vi "ConfigureDAQ.vi"(11 "DAQ Config Data":T1={"Vertical"={"Coupling"=0, "Offset (V)"=0.0, "Range (V)"=0.0, "Impedance"=0.0}, "Horizontal"={"Offset Time"=0.0, "Sample Time (S)"=0.0, "Sample Points"=0}, "Trigger\n"={"Lower Level (V)"=0.0, "Trigger Slope"=0, "Trigger Source"=0}, "Acquisition"={"Trigger Mode"=0, "Initiate Continuously"=0, "Acquire Type"=0, "Acquire Count"=1}, "Channel"=0, "Instrument Handle"=0, "Error"={"status"=FALSE, "code"=0, "source"=""}, "State"=0} {"State" items=["Enable"=1, "Disable"=0]; "Channel" items=["Input Channel 1", "Input Channel 2", "Input Channel 3", "Input Channel 4"]; "Acquisition"."Acquire Type" items=["Normal"=0, "Average"=1, "Envelope"=2, "Peak Detect"=3, "High Resolution"=4, "Fast"=5, "Equivalent Time"=16]; "Acquisition"."Initiate Continuously" items=["Continuously"=1, "Single Capture"=0]; "Acquisition"."Trigger Mode" items=["Auto", "Normal"]; "Trigger"."Trigger Source" items=["TTL0", "TTL1", "TTL2", "TTL3", "TTL4", "TTL5", "TTL6", "TTL7", "ECL0", "ECL1", "Input Channel 1", "Input Channel 2", "Input Channel 3", "Input Channel 4", "External Trigger Source", "STAR", "Manual Trigger", "Pattern"]; "Trigger"."Trigger Slope" items=["Rising Edge", "Falling Edge"]; "Horizontal"."Sample Time (S)" items=["0.5"=0.5, "0.4"=0.4, "0.25"=0.25, "0.2"=0.2, "0.1"=0.1, "0.05"=0.05, "0.04"=0.04, "0.025"=0.025, "0.02"=0.02, "0.01"=0.01, "0.005"=0.005, "0.004"=0.004, "0.0025"=0.0025, "0.002"=0.002, "0.001"=0.001, "5E-4"=0.0005, "4E-4"=0.0004, "2.5E-4"=0.00025, "2E-4"=0.0002, "1E-4"=0.0001, "5E-5"=5e-05, "4E-5"=4e-05, "2E-5"=2e-05, "5E-6"=5e-06, "1E-6"=1e-06, "5E-7"=5e-07, "1E-7"=1e-07, "5E-8"=5e-08, "1E-8"=1e-08]; "Vertical"."Impedance" items=["50 Ohm"=50.0, "1 MOhm"=1000000.0]; "Vertical"."Range (V)" items=["10"=10.0, "5"=5.0, "2"=2.0, "1"=1.0, "0.4"=0.4, "0.2"=0.2, "0.08"=0.08, "0.04"=0.04, "0.02"=0.02, "0.01"=0.01]; "Vertical"."Coupling" items=["AC", "DC"]}) -> (0 "error out":errorcluster, 3 "Instrument Handle Out":i32)   [LabVIEW 2023]
uses:
  TypeDefs/DataTypes/DAQConfig.ctl
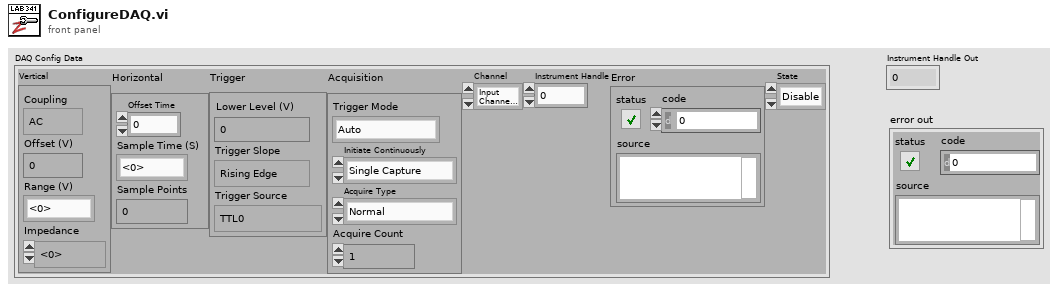
[diagram p1: front panel]
types:
  T1 = typedef "DAQConfig.ctl" = cluster{"Vertical":cluster{"Coupling":i32, "Offset (V)":dbl, "Range (V)":dbl, "Impedance":dbl}, "Horizontal":cluster{"Offset Time":dbl, "Sample Time (S)":dbl, "Sample Points":u32}, "Trigger\n":cluster{"Lower Level (V)":dbl, "Trigger Slope":i32, "Trigger Source":i32}, "Acquisition":cluster{"Trigger Mode":i32, "Initiate Continuously":i32, "Acquire Type":i32, "Acquire Count":i32}, "Channel":i32, "Instrument Handle":i32, "Error":errorcluster, "State":i32}
  T2 = cluster{"Lower Level (V)":dbl, "Trigger Slope":i32, "Trigger Source":i32}
  T3 = cluster{"Trigger Mode":i32, "Initiate Continuously":i32, "Acquire Type":i32, "Acquire Count":i32}
  T4 = cluster{"Coupling":i32, "Offset (V)":dbl, "Range (V)":dbl, "Impedance":dbl}
  T5 = cluster{"Offset Time":dbl, "Sample Time (S)":dbl, "Sample Points":u32}
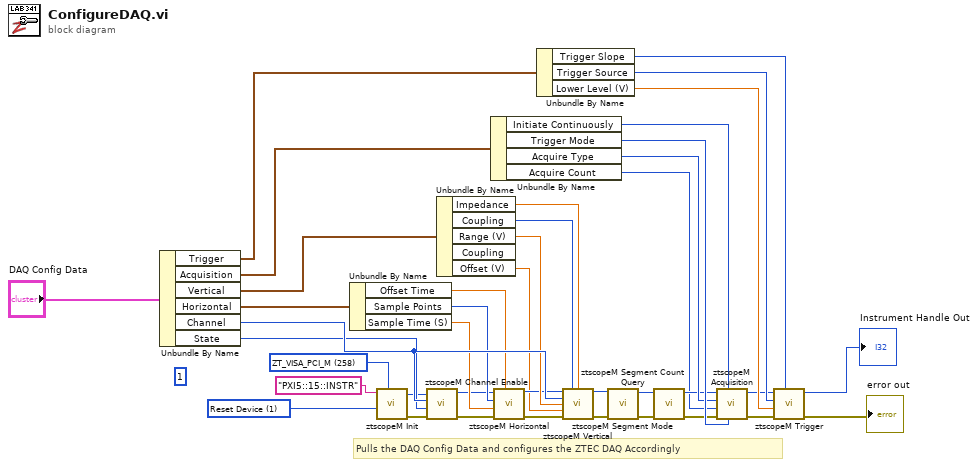
[diagram p0: block diagram]
diagram:
  w2 = u16 258 items=["ZT_MCLASS"=2, "ZT_LAN"=4, "ZT_VISA_PCI_M"=258, "ZT_VISA_M"=514] ("Comm Bus")
  (unwired) 1 ("Number of Cards to Search For")
  w16 = 1 items=["Reset Device"=1, "Don't Reset"=0] ("Reset")
  # "Pulls the DAQ Config Data and configures the ZTEC DAQ Accordingly"
  n1 = Unbundle By Name("DAQ Config Data") -> ("Trigger"=w37:T2, "Acquisition"=w33:T3, "Vertical"=w28:T4, "Horizontal"=w21:T5, "Channel"=w32:i32, "State"=w19:i32)
  n2 = Unbundle By Name(w21) -> ("Offset Time"=w26:dbl, "Sample Points"=w25:u32, "Sample Time (S)"=w24:dbl)
  n3 = call <instrlib>:"ztscopeM Init.vi"("Resource Name"="PXI5::15::INSTR", "Reset"=w16, "Comm Bus"=w2) -> ("Instrument Handle"=w14:i32, "error out"=w7:errorcluster)  [unwired: 5 in, 1 out]
  n4 = call <instrlib>:"ztscopeM Channel Enable.vi"("error in"=w7, "State"=w19, "Channel"=w32, "Instrument Handle In"=w14) -> ("error out"=w23:errorcluster, "Instrument Handle Out"=w22:i32)  [unwired: 6 in]
  n5 = Unbundle By Name(w28) -> ("Impedance"=w29:dbl, "Coupling"=w30:i32, "Range (V)"=w31:dbl, "Offset (V)"=w3:dbl)  [unwired: 1 out]
  n6 = Unbundle By Name(w33) -> ("Initiate Continuously"=w35:i32, "Trigger Mode"=w36:i32, "Acquire Type"=w34:i32, "Acquire Count"=w4:i32)
  n7 = call <instrlib>:"ztscopeM Horizontal.vi"("Offset Time"=w26, "error in"=w23, "Sample Time"=w24, "Sample Points"=w25, "Instrument Handle In"=w22) -> ("error out"=w15:errorcluster, "Instrument Handle Out"=w27:i32)  [unwired: 5 in]
  n8 = Unbundle By Name(w37) -> ("Trigger Slope"=w40:i32, "Trigger Source"=w39:i32, "Lower Level (V)"=w38:dbl)
  n9 = call <instrlib>:"ztscopeM Vertical.vi"("Instrument Handle In"=w27, "Coupling"=w30, "Impedance"=w29, "Channel"=w32, "Range"=w31, "Offset"=w3, "error in"=w15) -> ("Instrument Handle Out"=w6:i32, "error out"=w5:errorcluster)  [unwired: 7 in]
  n10 = call <instrlib>:"ztscopeM Segment Mode.vi"("error in"=w5, "Instrument Handle In"=w6) -> ("error out"=w11:errorcluster, "Instrument Handle Out"=w9:i32)  [unwired: 8 in]
  n11 = call <instrlib>:"ztscopeM Segment Count Query.vi"("error in"=w11, "Instrument Handle In"=w9) -> ("error out"=w10:errorcluster, "Instrument Handle Out"=w8:i32)  [unwired: 7 in, 1 out]
  n12 = call <instrlib>:"ztscopeM Acquisition.vi"("Trigger Mode"=w36, "Initiate Continuously"=w35, "error in"=w10, "Acquire Count"=w4, "Acquire Type"=w34, "Instrument Handle In"=w8) -> ("error out"=w12:errorcluster, "Instrument Handle Out"=w13:i32)  [unwired: 4 in]
  n13 = call <instrlib>:"ztscopeM Trigger.vi"("Slope"=w40, "error in"=w12, "Level"=w38, "Trigger Source"=w39, "Instrument Handle In"=w13) -> ("error out"=→"error out":errorcluster, "Instrument Handle Out"=→"Instrument Handle Out":i32)  [unwired: 4 in]
